vi "VI Tree.vi"   [LabVIEW 2010, in "Agilent DSO1000 Series.lvlib"]
doc: "This is the instrument driver for the Agilent DSO1000 series oscilloscope. The VI Tree displays all the user-callable VIs of the instrument driver in an organized table."
uses:
  <instrlib>/Agilent DSO1000 Series/Agilent DSO1000 Series.lvlib
  <instrlib>/Agilent DSO1000 Series/Public/Data/Read Waveform (Single).vi
  <instrlib>/Agilent DSO1000 Series/Public/Configure/Configure Trigger (Edge).vi
  <instrlib>/Agilent DSO1000 Series/Public/Configure/Configure Alternation Trigger (Edge).vi
panel:
  # "(c) 2009 National Instruments.  ALL RIGHTS RESERVED."
  # "SEE DIAGRAM\nFOR VI TREE."
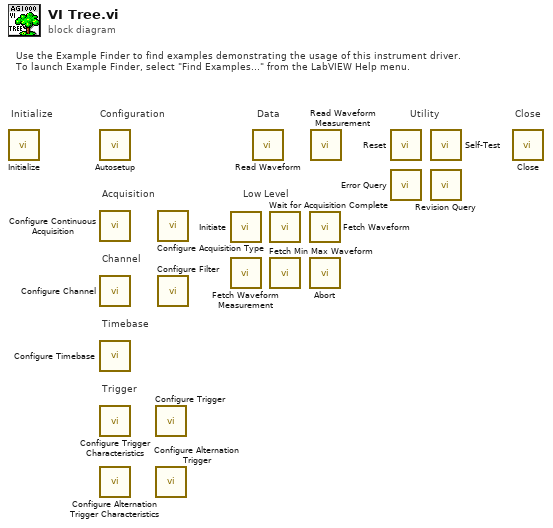
[diagram p0: block diagram]
diagram:
  # "Trigger"
  # "Timebase"
  # "Acquisition"
  # "Channel"
  # "Low Level"
  # "Use the Example Finder to find examples demonstrating the usage of this instrument driver.\nTo launch Example Finder, select \"Find Examples...\" from the LabVIEW Help menu."
  # "Configuration"
  # "Utility"
  # "Data"
  # "Close"
  # "Initialize"
  n1 = call <instrlib>:"Initialize.vi"() -> ()  [unwired: 10 in, 2 out]
  n2 = call <instrlib>:"Autosetup.vi"() -> ()  [unwired: 10 in, 2 out]
  n3 = call <instrlib>:"Configure Continuous Acquisition.vi"() -> ()  [unwired: 10 in, 2 out]
  n4 = call <instrlib>:"Configure Channel.vi"() -> ()  [unwired: 14 in, 2 out]
  n5 = call <instrlib>:"Configure Timebase.vi"() -> ()  [unwired: 10 in, 2 out]
  n6 = call <instrlib>:"Configure Trigger Characteristics.vi"() -> ()  [unwired: 10 in, 2 out]
  n7 = call <instrlib>:"Configure Alternation Trigger Characteristics.vi"() -> ()  [unwired: 14 in, 2 out]
  n8 = call-poly <instrlib>:"Configure Trigger.vi"() -> ()  [unwired: 14 in, 2 out]
  n9 = call-poly <instrlib>:"Configure Alternation Trigger.vi"() -> ()  [unwired: 14 in, 2 out]
  n10 = call <instrlib>:"Configure Acquisition Type.vi"() -> ()  [unwired: 10 in, 2 out]
  n11 = call <instrlib>:"Configure Filter.vi"() -> ()  [unwired: 10 in, 2 out]
  n12 = call <instrlib>:"Initiate.vi"() -> ()  [unwired: 10 in, 2 out]
  n13 = call <instrlib>:"Fetch Waveform Measurement.vi"() -> ()  [unwired: 9 in, 3 out]
  n14 = call-poly <instrlib>:"Read Waveform.vi"() -> ()  [unwired: 9 in, 3 out]
  n15 = call <instrlib>:"Wait for Acquisition Complete.vi"() -> ()  [unwired: 10 in, 2 out]
  n16 = call <instrlib>:"Fetch Min Max Waveform.vi"() -> ()  [unwired: 8 in, 4 out]
  n17 = call <instrlib>:"Fetch Waveform.vi"() -> ()  [unwired: 9 in, 3 out]
  n18 = call <instrlib>:"Abort.vi"() -> ()  [unwired: 10 in, 2 out]
  n19 = call <instrlib>:"Read Waveform Measurement.vi"() -> ()  [unwired: 9 in, 3 out]
  n20 = call <instrlib>:"Reset.vi"() -> ()  [unwired: 10 in, 2 out]
  n21 = call <instrlib>:"Error Query.vi"() -> ()  [unwired: 8 in, 4 out]
  n22 = call <instrlib>:"Self-Test.vi"() -> ()  [unwired: 8 in, 4 out]
  n23 = call <instrlib>:"Revision Query.vi"() -> ()  [unwired: 8 in, 4 out]
  n24 = call <instrlib>:"Close.vi"() -> ()  [unwired: 11 in, 1 out]
